vi "Valve Gearing (Read).vi"(6 "ISOBUS address":T3=-1 caption="ISOBUS address (-1)", 8 "error in":errorcluster, 11 "Mercury Reference In":T4) -> (0 "error out":errorcluster, 1 "Unit":T1, 2 "Gear":u32 caption="Valve Gearing", 3 "Mercury Reference Out":T4, 4 "Valid?":T2)   [LabVIEW 2015, in "Mercury iXX.lvlib" / "Auxiliary.lvlib"]
doc: "Read the current configuration for the valve gearing setting."
uses:
  Auxiliary.lvlib
  Controls/Mercury Reference.ctl
  Controls/Comms Transport Layer.ctl
  private/Controls/Query Dynamic Reference.ctl
  Controls/ISOBus Address.ctl
  Controls/Is Valid LED.ctl
  Controls/Unit String.ctl
  private/Controls/Command Verbs.ctl
  Mercury iXX.lvlib
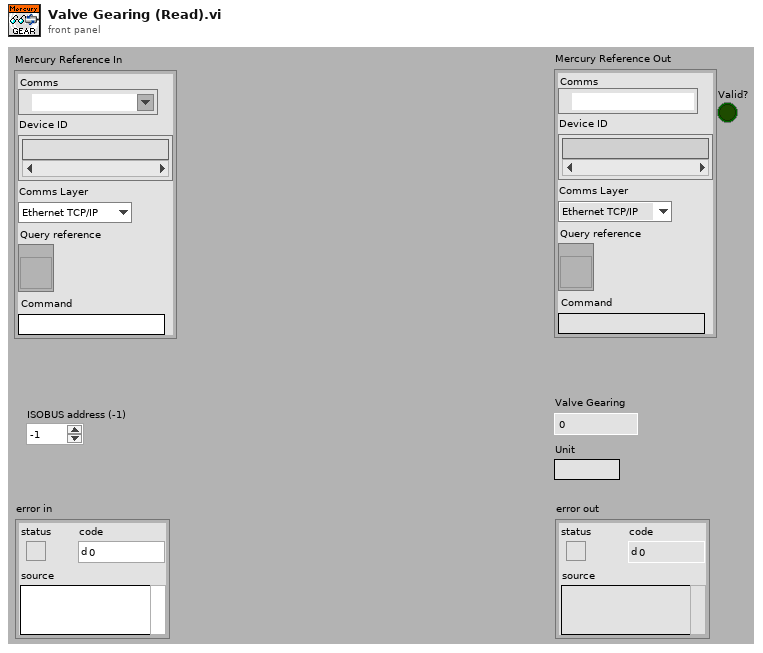
[diagram p1: front panel]
types:
  T1 = typedef "Mercury iXX.lvlib/Unit String.ctl" = string
  T2 = typedef "Mercury iXX.lvlib/Is Valid LED.ctl" = bool
  T3 = typedef "Mercury iXX.lvlib/ISOBus Address.ctl" = i32
  T4 = typedef "Mercury iXX.lvlib/Mercury Reference.ctl" = cluster{"Comms":refnum<visa-resource-name>, "Device ID":string[], "Comms Layer":T5, "Command":string, "Query reference":T6}
  T5 = typedef "Mercury iXX.lvlib/Comms Transport Layer.ctl" = enum16{"Ethernet TCP/IP", "USB", "ISOBus - RS-232", "GPIB"}
  T6 = typedef "Mercury iXX.lvlib/Query Dynamic Reference.ctl" = refnum<vi>
  T7 = typedef "Mercury iXX.lvlib/Command Verbs.ctl" = string
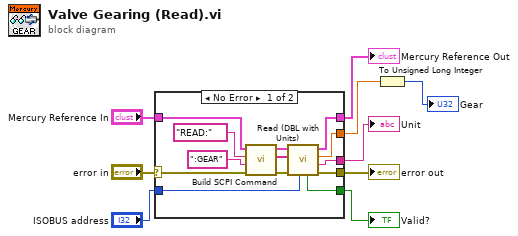
[diagram p0: block diagram]
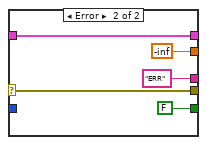
[diagram p2: hidden frame]
diagram:
  n1 = case shown="No Error" "error in" {
    selector: "error in" -> [w21 w27]
    tunnel: "Mercury Reference In" -> [w22 w26]
    tunnel: [w15 w26] -> w8
    tunnel: [w10 w27] -> w5
    tunnel: "ISOBUS address" -> [w12 _]
    tunnel: [w13 T2 FALSE ("Valid?")] -> w4
    tunnel: [w14 -inf] -> w3
    tunnel: [w16 T1 "ERR" ("Unit")] -> w2
    frame No Error {
      n2 = call "Build SCPI Command.vi"("error in"=w21, "Noun(s)"=":GEAR" ("Command"), "Verb"=T7 "READ:", "Mercury Reference In"=w22) -> ("error out"=w18:errorcluster, "SCPI Message(s)"=w11:string[], "Mercury Reference Out"=w17:T4)  [unwired: 5 out]
      n3 = call "Read (DBL with Units).vi"("ISOBUS address"=w12, "error in"=w18, "SCPI Message(s)"=w11, "Mercury Reference In"=w17) -> ("error out"=w10:errorcluster, "Unit"=w16:T1, "Data (Dbl)"=w14:dbl, "Mercury Reference Out"=w15:T4, "Valid?"=w13:T2)  [unwired: 3 out]
    }
    frame Error {
    }
  }
  "Mercury Reference Out" <- w8
  "error out" <- w5
  "Valid?" <- w4
  "Unit" <- w2
  n4 = To Unsigned Long Integer(number=w3) -> (unsigned 32bit integer=→"Gear":u32)
